vi "test_clipboard.vi"() -> ()   [LabVIEW 2013]
uses:
  System.Windows.Forms
panel:
  out "error out":errorcluster
  out "new picture":picture
  in  "PictureBox":refnum<k24>(container)
  out "Waveform Chart":dbl(graph)
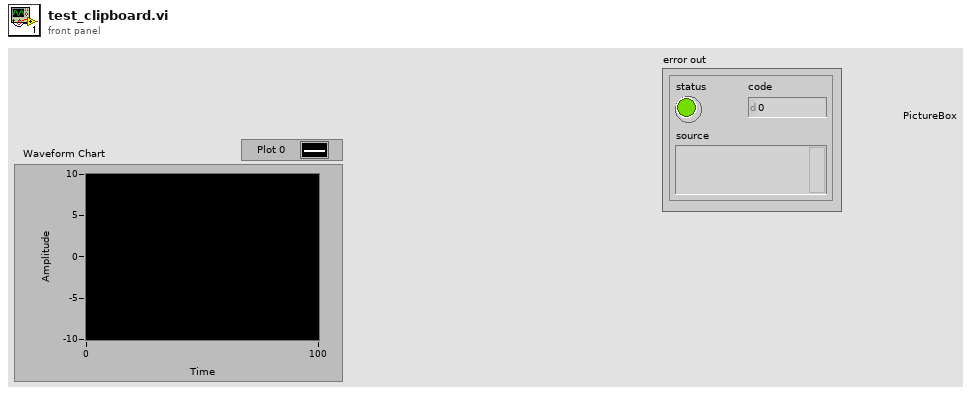
[diagram p1: front panel]
types:
  T1 = typedef "imagedata.ctl" = cluster{"image type":i32, "image depth":i32, "image":u8[], "mask":u8[], "colors":u32[], "Rectangle":cluster{"left":i16, "top":i16, "right":i16, "bottom":i16}}
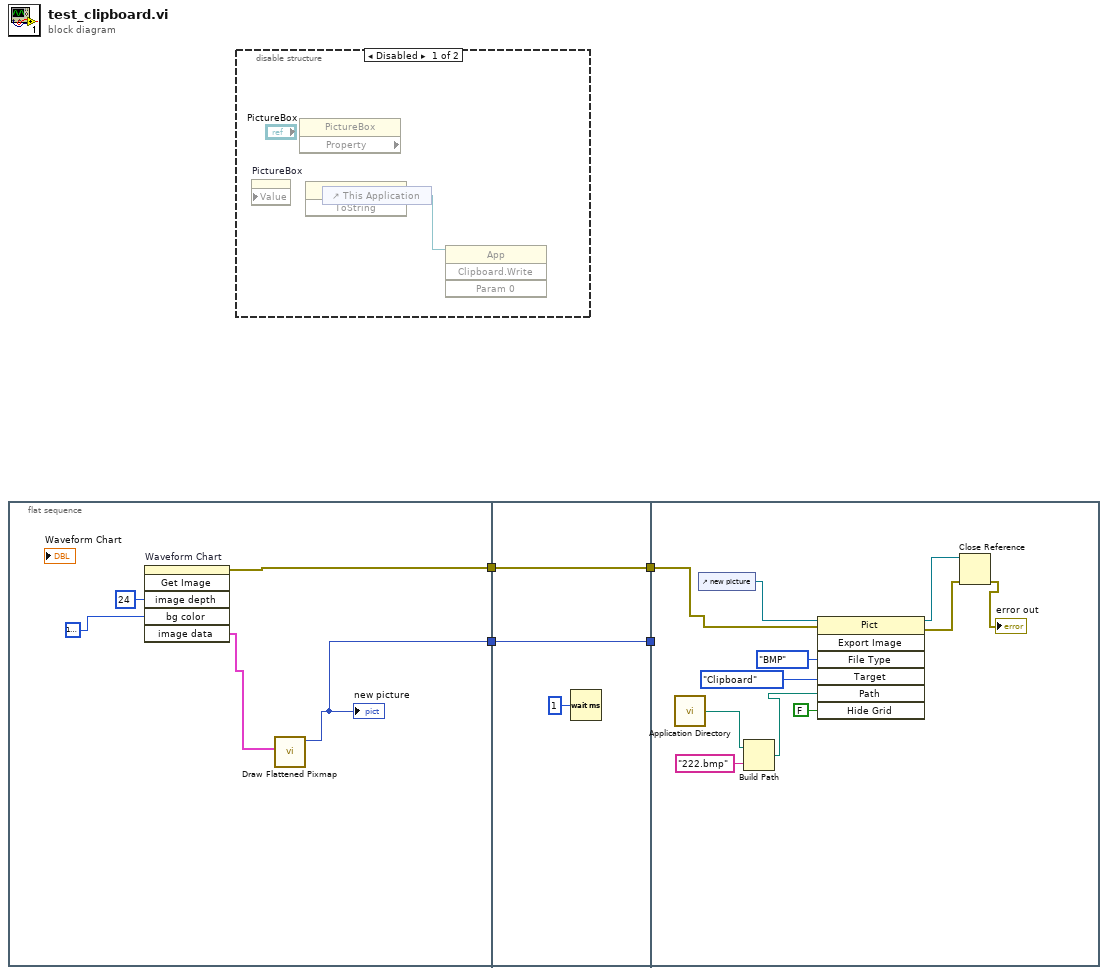
[diagram p0: block diagram]
diagram:
  n1 = flat-sequence {
    tunnel: [w6] -> w4
    tunnel: [w5] -> w2
    tunnel: w4 -> [w12]
    tunnel: [w12] -> w3
    tunnel: w2 -> [w11]
    tunnel: [w11] -> w1
    tunnel: w3 -> [_]
    tunnel: w1 -> [w20]
    frame #0 {
      n2 = invoke on="Waveform Chart" class="WFChart (strict)" method="Get Image"("image depth"=24 ("Image Depth"), "bg color"=u32 16777216) -> (error out=w5:errorcluster, "image data"=w7:T1)  [unwired: 4 in, 4 out]
      n3 = call <vilib>:"Draw Flattened Pixmap.vi"("image data"=w7) -> ("new picture"=w6:picture)  [unwired: 8 in]
      "new picture" <- w6
    }
    frame #1 {
      n4 = Wait (ms)(milliseconds to wait=u32 1) -> ()  [unwired: 1 out]
    }
    frame #2 {
      n5 = call <vilib>:"Application Directory.vi"() -> ("Application Directory"=w18:path)
      n6 = control-ref of="new picture"() -> (w19:refnum<vi>)
      n7 = Build Path(base path=w18, name or relative path="222.bmp") -> (appended path=w16:path)
      n8 = invoke class="Pict" method="Export Image"(reference=w19, error in=w20, "File Type"=enum32{"BMP", "EPS", "EMF", "PICT"}."BMP", "Target"=enum32{"File", "Clipboard"}."Clipboard", "Path"=w16, "Hide Grid"=FALSE ("Always Overwrite")) -> (reference out=w15:refnum<vi>, error out=w14:errorcluster)  [unwired: 1 in, 5 out]
      n9 = Close Reference(reference=w15, error in (no error)=w14) -> (error out=→"error out":errorcluster)
    }
  }
  n10 = disable-structure shown="Disabled" {
    frame Disabled {
      n11 = property on="PictureBox" class="AXCont" props=["Value"]() -> ()  [unwired: 3 in, 2 out]
      n12 = property class="PictureBox" props=[]() -> ()  [unwired: 2 in, 3 out]
      n13 = invoke class="PictureBox" method="ToString"() -> ()  [unwired: 3 in, 3 out]
      n14 = control-ref of="This Application"() -> (w24:refnum<vi>)
      n15 = invoke class="App" method="Clipboard.Write"(reference=w24) -> ()  [unwired: 3 in, 4 out]
    }
    frame Enabled {
    }
  }
